vi "Read Multiple Event Registration.vi"(6 "number of event structures":u16=2, 10 "Channel":T1) -> (2 "Event Registration Refnums":refnum<event-registration>[](array[refnum]))   [LabVIEW 2020, in "Event Messenger Priority.lvlib"]
doc: "<p>Reads multiple <a href=\"nihelplauncher://docs/csh?context=lvcore_lvconcepts_using_events_in_labview\">event registration</a> refnums for an Event Messenger Priority<a href=\"nihelplauncher://docs/csh?context=lvcore_lvconcepts_channel_wires_intro\">channel</a> and makes the refnums available to one or more <a href=\"nihelplauncher://docs/csh?context=lvcore_glang_event_structure\">Event structures</a>.</p>"
uses:
  Event Messenger Priority.lvlib
  ChannelOp.ctl
  ))Channel.ctl
  Element.ctl
  Event Data.ctl
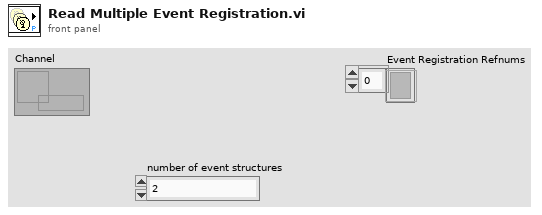
[diagram p1: front panel]
types:
  T1 = typedef "Event Messenger Priority.lvlib/))Channel.ctl" = refnum<queue>
  T2 = typedef "Event Messenger Priority.lvlib/ChannelOp.ctl" = enum16{"init", "write", "register", "replicate", "probe"}
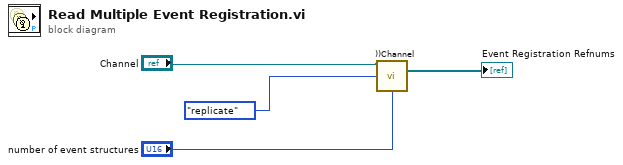
[diagram p0: block diagram]
diagram:
  n1 = call "))Channel.vi"("channel out"="Channel", "channelOp"=ChannelOp."replicate", "# event structures"="number of event structures") -> ("Event Registration Refnum"=→"Event Registration Refnums":refnum<event-registration>[])  [unwired: 8 in, 4 out]
